vi "Write Work Space.vi"(3 "FP":refnum<class "FP.lvclass">, 4 "WkSpace":T1) -> (5 "FP Out":refnum<class "FP.lvclass">)   [LabVIEW 2023, in "FP.lvclass"]
uses:
  FP.lvclass
  <vilib>/Utility/miscctls.llb/LVRectTypeDef.ctl
  FP.lvclass/FP.ctl
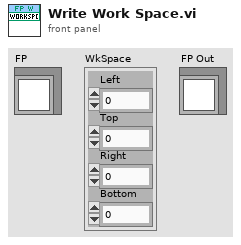
[diagram p1: front panel]
types:
  T1 = typedef "LVRectTypeDef.ctl" = cluster{"Left":i16, "Top":i16, "Right":i16, "Bottom":i16}
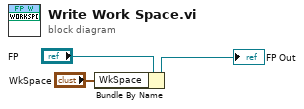
[diagram p0: block diagram]
diagram:
  n1 = Bundle By Name(cluster="FP", "WkSpace"="WkSpace") -> (→"FP Out":refnum<class "FP.lvclass">)
